vi "AggregateReports.vi"(6 "Additional In":T1 {"Synx" format="%#_4g"}, 11 "Aggregated In":T1 {"Synx" format="%#_4g"}) -> (3 "Aggregated Out":T1 {"Synx" format="%#_4g"})   [LabVIEW 2017, in "Bus_class.lvlib" / "Bus.lvclass"]
uses:
  Bus.lvclass
  Modules/EventPlugins/EventPluginBaseClass/TypeDefs/clEvtReportArray.ctl
  Modules/EventPlugins/EventPluginBaseClass/TypeDefs/clEvtReport.ctl
  Modules/EventPlugins/EventPluginBaseClass/EventPluginBaseClass.lvclass
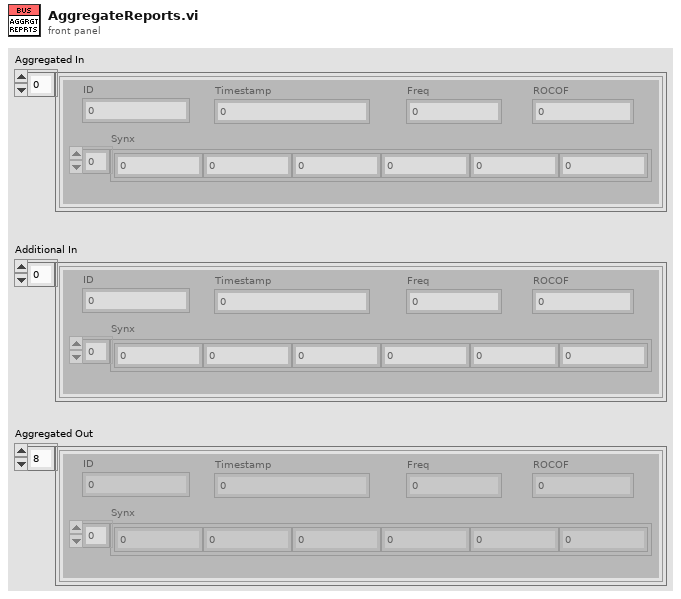
[diagram p1: front panel]
types:
  T1 = typedef "EventPlugins.lvlib/EventPluginBaseClass.lvclass/clEvtReportArray.ctl" = T2[]
  T2 = typedef "EventPlugins.lvlib/EventPluginBaseClass.lvclass/clEvtReport.ctl" = cluster{"Timestamp":dbl, "Synx":cdb[], "Freq":dbl, "ROCOF":dbl, "ID":i16}
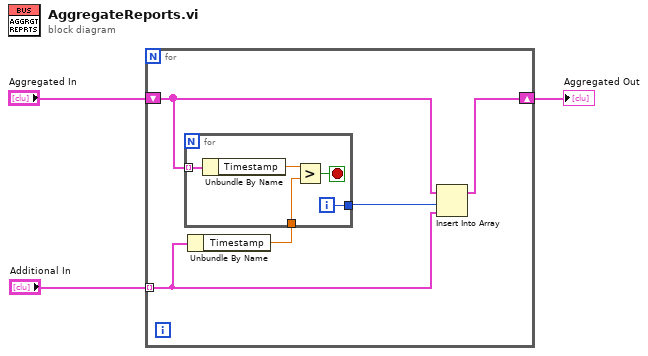
[diagram p0: block diagram]
diagram:
  n1 = for {
    tunnel: "Additional In" -> [w6] mode=indexing
    shift-right: [w4] -> w1
    shift-left: "Aggregated In" -> [w5]
    n2 = Unbundle By Name(w6) -> ("Timestamp"=w8:dbl)
    n3 = for {
      tunnel: w5 -> [w13] mode=indexing
      tunnel: w8 -> [w11]
      tunnel: [w9] -> w7
      i -> [w9]
      stop <- w10 stop-if-true
      n4 = Unbundle By Name(w13) -> ("Timestamp"=w12:dbl)
      n5 = Greater?(x=w12, y=w11) -> (0:w10:bool)
    }
    n6 = Insert Into Array(array=w5, index=w7, new element=w6) -> (w4:T1)
  }
  "Aggregated Out" <- w1
